vi "Read Config VI.vi"(8 "error in (no error)":errorcluster, 11 "Plugin in":refnum<class "Plugin.lvclass">) -> (0 "error out":errorcluster, 2 "VI Refnum":refnum<vi>, 3 "Plugin out":refnum<class "Plugin.lvclass">)   [LabVIEW 2015, in "Plugin.lvclass"]
uses:
  Plugin.lvclass
  Default Config VI.vi
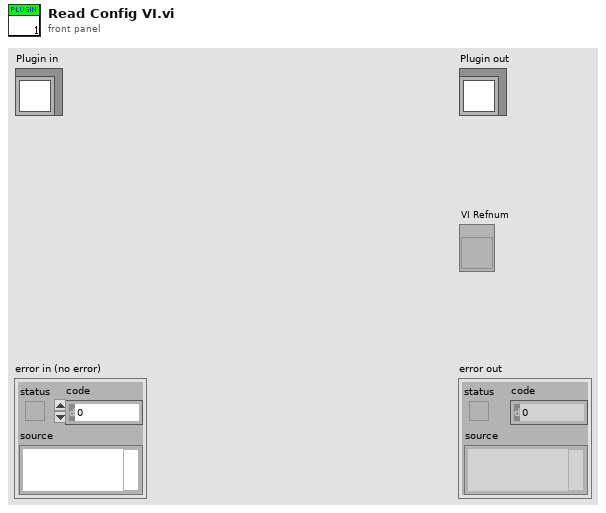
[diagram p1: front panel]
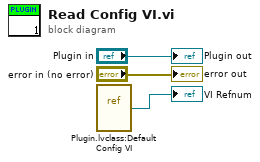
[diagram p0: block diagram]
diagram:
  n1 = vi-ref "Plugin.lvclass:Default Config VI.vi"() -> (→"VI Refnum":refnum<vi>)
  "error out" <- "error in (no error)"
  "Plugin out" <- "Plugin in"
